vi "Get Module Configuration Revision from Identifier.vi"(8 "error in":errorcluster, 10 "module identifier":string, 11 "routing and faulting in":T1 format="%.0x") -> (0 "error out":errorcluster, 2 "configuration revision":u32, 3 "routing and faulting out":T1 format="%.0x")   [LabVIEW 2020, in "Routing and Faulting Scripting.lvlib"]
uses:
  Routing and Faulting Scripting.lvlib
  <vilib>/NI VeriStand/Custom Device API/Custom Device Item Ref.ctl
  NationalInstruments.VeriStand.SystemStorage
  <vilib>/NI VeriStand/Custom Device API/Custom Device API.lvlib
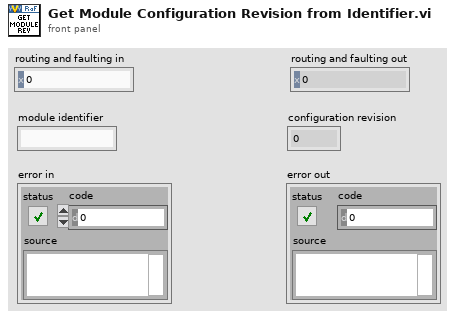
[diagram p1: front panel]
types:
  T1 = typedef "Custom Device API.lvlib/Custom Device Item Ref.ctl" = u64
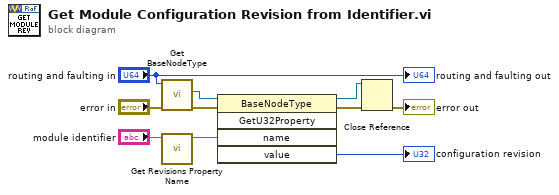
[diagram p0: block diagram]
diagram:
  n1 = call "Get BaseNodeType.vi"("error in"="error in", "item in"="routing and faulting in") -> ("error out"=w6:errorcluster, "BaseNodeType"=w5:refnum<k24>)  [unwired: 7 in, 1 out]
  n2 = call "Get Revisions Property Name.vi"("module identifier"="module identifier") -> ("module revision property name"=w10:string)  [unwired: 10 in]
  n3 = invoke class="BaseNodeType" method="GetU32Property"(reference=w5, error in=w6, "name"=w10) -> (reference out=w2:refnum<k24>, error out=w8:errorcluster, "value"=→"configuration revision":u32)  [unwired: 2 in, 2 out]
  n4 = Close Reference(reference=w2, error in (no error)=w8) -> (error out=→"error out":errorcluster)
  "routing and faulting out" <- "routing and faulting in"
